vi "ENPH354_A4Q3.vi"() -> ()   [LabVIEW 2020]
uses:
  bb56ae38-73f5-4382-81c7-8fb4f485a9da.vi
  <vilib>/Array/Sort 2D Array - Pop Stack.vi
  <vilib>/Array/Sort 2D Array - Push Stack.vi
  bb56ae38-73f5-4382-81c7-8fb4f485a9da.vi/269d4b3b-47f5-49e3-8884-44851e4dd9d5.vi
  bb56ae38-73f5-4382-81c7-8fb4f485a9da.vi/6d99389c-673d-4efb-bf33-19b32bcf4cf8.vi
  <vilib>/Utility/file.llb/Read Delimited Spreadsheet (DBL).vi
  <vilib>/Analysis/NI_AALPro.lvlib
panel:
  in  "Save Reduced Fitted Data":path
  in  "Save Reduced Data":path
  out "LSLF Intercept [mA/mW]":dbl
  out "LSLF Slope [mA/mW/nm]":dbl
  out "Absolute Spectra Sensitivity \nData Sorted and Below 700nm":dbl[][](array[numeric])
  out "Reduced and Fitted Data\nAbsolute Spectra Sensitivity Below 700nm":cluster{dbl[], "Best Linear Fit":dbl[]}[](graph)
  out "Sorted and Converted Data\nAbsolute Spectra Sensitivity":cluster{"X":dbl[], "Y":dbl[]}[](graph)
  out "Absolute Spectra Sensitivity\nSorted":dbl[][](array[numeric])
  out "Original Data\nRelative Spectra Sensitivity":cluster{"X":dbl[], "Y":dbl[]}[](graph)
  out "Relative Spectra Sensitivity":dbl[][](array[numeric])
  in  "PhotodiodeSensData":path
  # "ENPH354 Assignment 4 Q3"
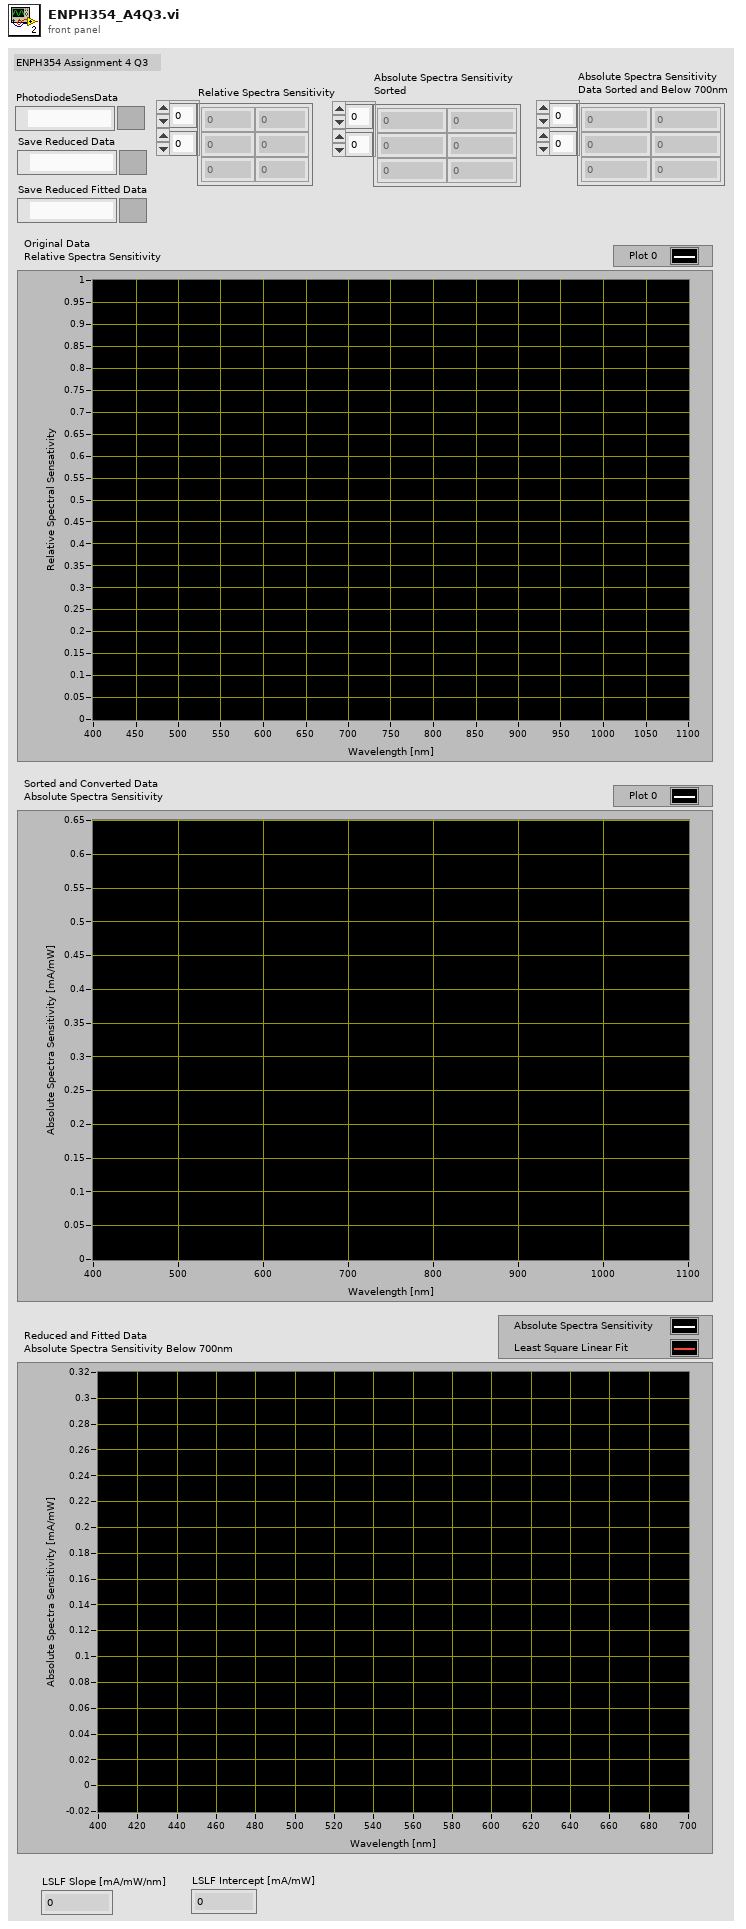
[diagram p1: front panel]
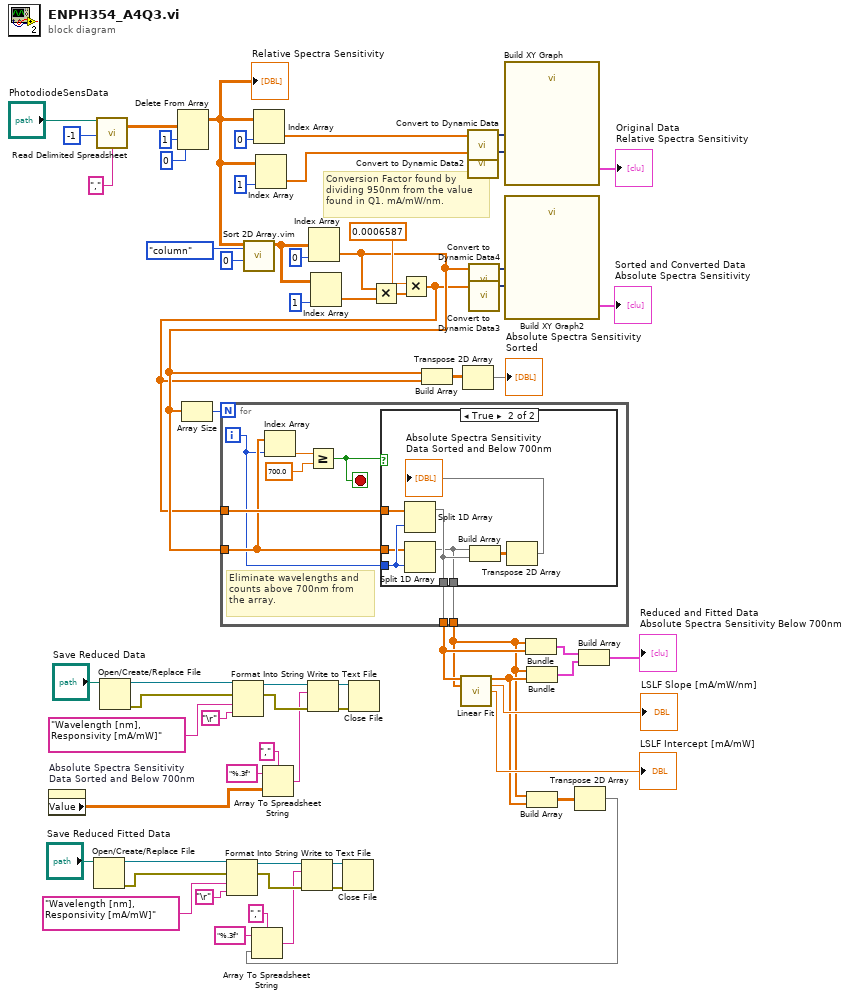
[diagram p0: block diagram]
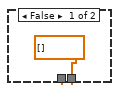
[diagram p2: hidden frame]
diagram:
  # "Conversion Factor found by\ndividing 950nm from the value\nfound in Q1. mA/mW/nm."
  n1 = property on="Absolute Spectra Sensitivity \nData Sorted and Below 700nm" class="Arr (strict)"() -> ("Value"=w18:dbl[][])  [unwired: 2 in, 2 out]
  n2 = Open/Create/Replace File(file path (use dialog)="Save Reduced Fitted Data") -> (refnum out=w17:refnum<file>, error out=w14:errorcluster)  [unwired: 5 in, 1 out]
  n3 = call-poly <vilib>:"Read Delimited Spreadsheet.vi"("file path (dialog if empty)"="PhotodiodeSensData", "number of rows (all:-1)"=-1, "delimiter (\\t)"="," ("delimiter (\\t)")) -> ("all rows"=w62:dbl[][])  [unwired: 7 in, 5 out]
  n4 = Open/Create/Replace File(file path (use dialog)="Save Reduced Data") -> (refnum out=w30:refnum<file>, error out=w27:errorcluster)  [unwired: 5 in, 1 out]
  n5 = Delete From Array(array=w62, length=1, index (row)=0) -> (array with subset deleted=w52:dbl[][])  [unwired: 1 in, 1 out]
  "Relative Spectra Sensitivity" <- w52
  n6 = Format Into String(initial string=w17, error in=w14, "Wavelength [nm], Responsivity [mA/mW]", "\r") -> (resulting string=w16:refnum<file>, error out=w13:errorcluster)  [unwired: 1 in]
  n7 = Format Into String(initial string=w30, error in=w27, "Wavelength [nm], Responsivity [mA/mW]", "\r") -> (resulting string=w29:refnum<file>, error out=w26:errorcluster)  [unwired: 1 in]
  n8 = call "Sort 2D Array.vim"("index"=0, "dimension to index (column)"=enum16{"column", "row"}."column", "2D array"=w52) -> ("sorted 2D array"=w50:dbl[][])  [unwired: 7 in, 1 out]
  n9 = Index Array(array=w52, index (col)=0) -> (element=w57:dbl[])  [unwired: 1 in]
  n10 = Index Array(array=w52, index (col)=1) -> (element=w49:dbl[])  [unwired: 1 in]
  n11 = Array To Spreadsheet String(delimiter (Tab)=",", array=w18, 3:"%.3f" ("format string")) -> (spreadsheet string=w22:string)
  n12 = Write to Text File(file (use dialog)=w29, text=w22, error in=w26) -> (refnum out=w28:refnum<file>, error out=w25:errorcluster)  [unwired: 1 in, 1 out]
  n13 = Index Array(array=w50, index (col)=0) -> (element=w32:dbl[])  [unwired: 1 in]
  n14 = Array Size(array=w32) -> (size(s)=w38:i32)
  n15 = Index Array(array=w50, index (col)=1) -> (element=w45:dbl[])  [unwired: 1 in]
  n16 = Close File(refnum=w28, error in=w25) -> ()  [unwired: 2 out]
  n17 = Multiply(x=w32, y=w45) -> (x*y=w44:dbl[])
  n18 = Multiply(x=0.0006587 ("y"), y=w44) -> (x*y=w31:dbl[])
  n19 = for {
    N: w38 -> [_]
    tunnel: w31 -> [w70]
    tunnel: w32 -> [w69]
    tunnel: [w67] -> w37
    tunnel: [w66] -> w3
    i -> [w68]
    stop <- w71 stop-if-true
    # "Eliminate wavelengths and \ncounts above 700nm from\nthe array."
    n20 = Index Array(array=w69, index=w68) -> (element=w73:dbl)
    n21 = Greater Or Equal?(x=w73, y=700.0) -> (x >= y?=w71:bool)
    n22 = case shown="True" w71 {
      tunnel: w70 -> [_ w81]
      tunnel: w69 -> [_ w79]
      tunnel: w68 -> [_ w80]
      tunnel: [w74 w77] -> w67
      tunnel: [w74 w76] -> w66
      frame False {
        w74 = dbl[] []
      }
      frame True {
        n23 = Split 1D Array(array=w81, index=w80) -> (first subarray=w77:dbl[])  [unwired: 1 out]
        n24 = Split 1D Array(array=w79, index=w80) -> (first subarray=w76:dbl[])  [unwired: 1 out]
        n25 = Build Array(w76, w77) -> (w78:dbl[][])
        n26 = Transpose 2D Array(2D array=w78) -> (transposed array=→"Absolute Spectra Sensitivity \nData Sorted and Below 700nm":dbl[][])
      }
    }
  }
  n27 = Build Array(w32, w31) -> (w40:dbl[][])
  n28 = call <vilib>:"Linear Fit.vi"("Y"=w37, "X"=w3) -> ("Best Linear Fit"=w4:dbl[], "slope"=→"LSLF Slope [mA/mW/nm]":dbl, "intercept"=→"LSLF Intercept [mA/mW]":dbl)  [unwired: 9 in, 2 out]
  n29 = Transpose 2D Array(2D array=w40) -> (transposed array=→"Absolute Spectra Sensitivity\nSorted":dbl[][])
  n30 = call "Convert to Dynamic Data"("Array"=w57) -> ("Dynamic Data Type"=w56:dynamicdata)  [unwired: 3 in]
  n31 = call "Convert to Dynamic Data2"("Array"=w49) -> ("Dynamic Data Type"=w55:dynamicdata)  [unwired: 3 in]
  n32 = call "Convert to Dynamic Data4"("Array"=w32) -> ("Dynamic Data Type"=w41:dynamicdata)  [unwired: 3 in]
  n33 = call "Convert to Dynamic Data3"("Array"=w31) -> ("Dynamic Data Type"=w42:dynamicdata)  [unwired: 3 in]
  n34 = call "Build XY Graph"("Y Input"=w55, "X Input"=w56) -> ("XY Graph"=→"Original Data\nRelative Spectra Sensitivity":cluster{"X":dbl[], "Y":dbl[]}[])  [unwired: 8 in, 1 out]
  n35 = call "Build XY Graph2"("Y Input"=w42, "X Input"=w41) -> ("XY Graph"=→"Sorted and Converted Data\nAbsolute Spectra Sensitivity":cluster{"X":dbl[], "Y":dbl[]}[])  [unwired: 8 in, 1 out]
  n36 = Bundle(w3, w37) -> (w36:cluster{dbl[], dbl[]})  [unwired: 1 in]
  n37 = Bundle(w3, "Best Linear Fit"=w4) -> (w5:cluster{dbl[], "Best Linear Fit":dbl[]})  [unwired: 1 in]
  n38 = Build Array(w3, w4) -> (w2:dbl[][])
  n39 = Transpose 2D Array(2D array=w2) -> (transposed array=w1:dbl[][])
  n40 = Array To Spreadsheet String(delimiter (Tab)=",", array=w1, 3:"%.3f" ("format string")) -> (spreadsheet string=w9:string)
  n41 = Write to Text File(file (use dialog)=w16, text=w9, error in=w13) -> (refnum out=w15:refnum<file>, error out=w12:errorcluster)  [unwired: 1 in, 1 out]
  n42 = Close File(refnum=w15, error in=w12) -> ()  [unwired: 2 out]
  n43 = Build Array(w36, w5) -> (→"Reduced and Fitted Data\nAbsolute Spectra Sensitivity Below 700nm":cluster{dbl[], "Best Linear Fit":dbl[]}[])
